vi "back_go_160607_85.vi"() -> ()   [LabVIEW 2015]
uses:
  <vilib>/NXT/Block Support/NXT_InputPort.ctl
  <vilib>/NXT/Block Support/NXT_OutputPort.ctl
  <vilib>/NXT/Dual Mode Library/Sensors/Light_On.vi
  <vilib>/NXT/Dual Mode Library/Sensors/Touch_Pressed.vi
  <vilib>/NXT/NXTIO Xnodes/NXTIONodeSubVIs/NXTMoveMotors.vi
  <vilib>/NXT/Dual Mode Library/Sensors/Sonar_cm.vi
  <vilib>/NXT/Dual Mode Library/Waits/Wait_Num.vi
  <vilib>/NXT/Subs/LVHSConnector.ctl
  <vilib>/NXT/NXTIO Xnodes/AddressXNode/NXTIOAddress.xnode
  <vilib>/NXT/NXTIO Xnodes/NXTIOXNode/NXTIO.xnode
  <vilib>/NXT/LegoClasses/BrickReference/BrickReference.lvclass
panel:
  in  "turn lefttC 2":i8=75
  in  "turn lefttB 2":i8=75
  in  "Go-ahead":i8=75
  out "check destance":i16(slide) scale=0.0..100.0
  in  "turn rightC":i8=75
  in  "turn rightB":i8=75
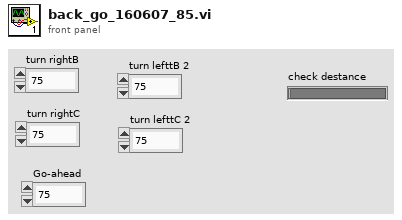
[diagram p1: front panel]
types:
  T1 = typedef "NXT_OutputPort.ctl" = u8
  T2 = typedef "NXT_InputPort.ctl" = u32
  T3 = typedef "LVHSConnector.ctl" = refnum<class "BrickReference.lvclass">
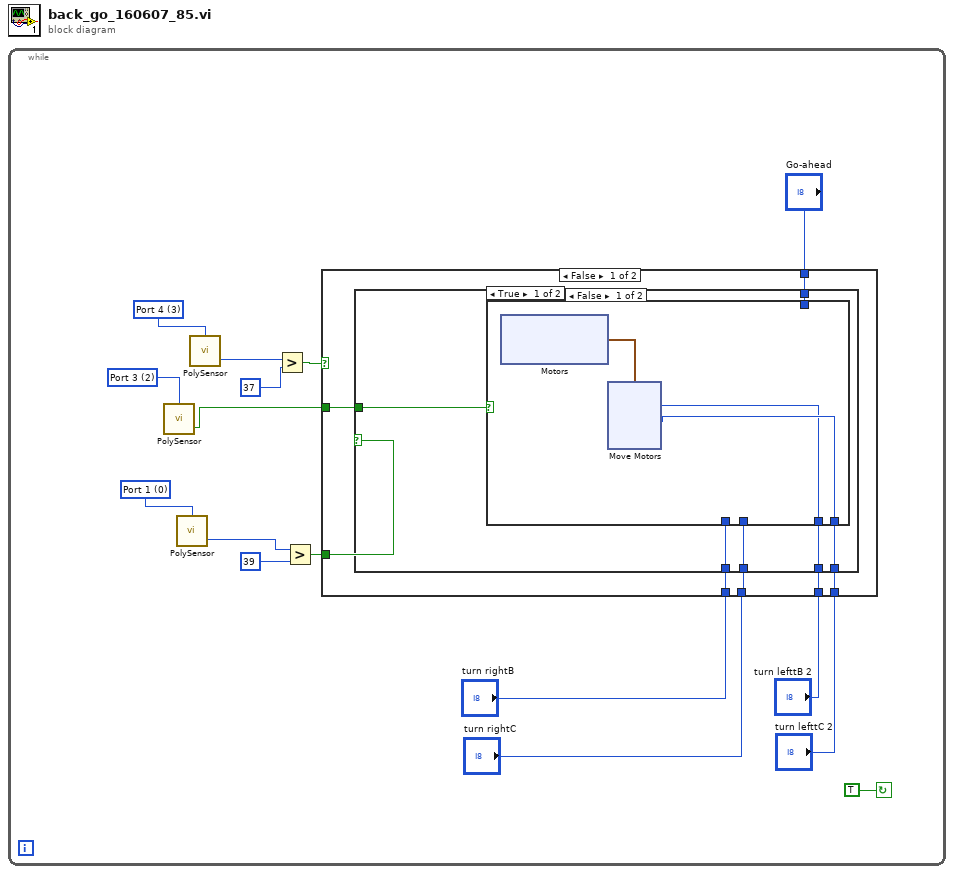
[diagram p0: block diagram]
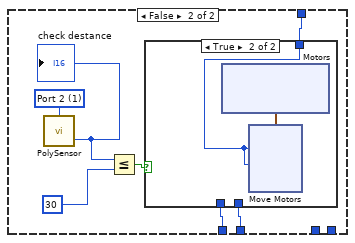
[diagram p2: hidden frame]
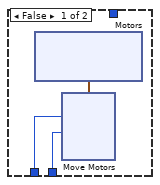
[diagram p3: hidden frame]
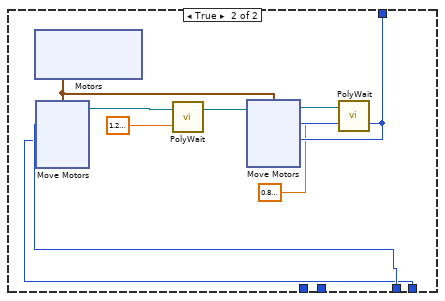
[diagram p4: hidden frame]
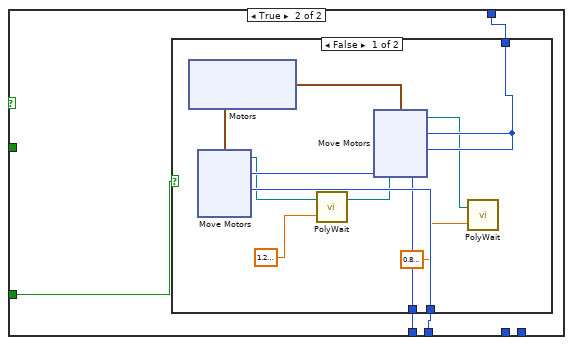
[diagram p5: hidden frame]
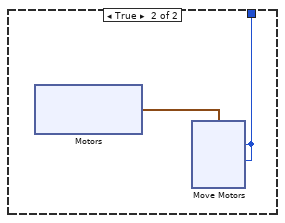
[diagram p6: hidden frame]
diagram:
  n1 = while {
    stop <- TRUE continue-if-true
    w1 = T2 2 items=["Port 1", "Port 2", "Port 3", "Port 4"] ("Port (Port 1)")
    w12 = T2 3 items=["Port 1", "Port 2", "Port 3", "Port 4"] ("Port (Port 3)")
    w11 = T2 0 items=["Port 1", "Port 2", "Port 3", "Port 4"] ("Port (Port 3)")
    n2 = call-poly <vilib>:"PolySensor.vi"("Port (Port 1)"=w1) -> ("Yes / No"=w2:bool)  [unwired: 2 in, 1 out]
    n3 = call-poly <vilib>:"PolySensor.vi"("Port (Port 3)"=w11) -> ("Scaled Value"=w13:i16)  [unwired: 2 in, 1 out]
    n4 = call-poly <vilib>:"PolySensor.vi"("Port (Port 3)"=w12) -> ("Scaled Value"=w15:i16)  [unwired: 2 in, 1 out]
    n5 = Greater?(x=w15, y=i16 37) -> (0:w10:bool)
    n6 = Greater?(x=w13, y=i16 39) -> (0:w9:bool)
    n7 = case shown="False" w10 {
      tunnel: w9 -> [w23 w101]
      tunnel: "turn rightB" -> [w22 w100]
      tunnel: "turn rightC" -> [w21 w99]
      tunnel: "Go-ahead" -> [w20 w98]
      tunnel: "turn lefttB 2" -> [w19 _]
      tunnel: "turn lefttC 2" -> [w18 _]
      tunnel: w2 -> [w17 _]
      frame False {
        n8 = case shown="False" w23 {
          tunnel: w22 -> [w29 _]
          tunnel: w21 -> [w28 _]
          tunnel: w20 -> [w27 w76]
          tunnel: w19 -> [w25 w80]
          tunnel: w18 -> [w24 w79]
          tunnel: w17 -> [w26 _]
          frame False {
            n9 = case shown="True" w26 {
              tunnel: w29 -> [_ w48]
              tunnel: w28 -> [_ w47]
              tunnel: w27 -> [_ w42]
              tunnel: w25 -> [w30 _]
              tunnel: w24 -> [w31 _]
              frame True {
                n10 = xnode "Motors"() -> ("Motor"=w32:cluster{"Port":T1, "Port":T1})
                n11 = xnode "Move Motors"("Power/Speed 2"=w31, "Power/Speed 1"=w30, "Motors"=w32) -> ()  [unwired: 1 in, 1 out]
              }
              frame False {
                w45 = T2 1 items=["Port 1", "Port 2", "Port 3", "Port 4"] ("Port (Port 4)")
                n12 = call-poly <vilib>:"PolySensor.vi"("Port (Port 4)"=w45) -> ("Distance (cm)"=w46:i16)  [unwired: 2 in, 1 out]
                "check destance" <- w46
                n13 = Less Or Equal?(x=w46, y=i16 30) -> (x <= y?=w43:bool)
                n14 = case shown="True" w43 {
                  tunnel: w48 -> [w50 _]
                  tunnel: w47 -> [w49 _]
                  tunnel: w42 -> [_ w61]
                  frame False {
                    n15 = xnode "Motors"() -> ("Motor"=w51:cluster{"Port":T1, "Port":T1})
                    n16 = xnode "Move Motors"("Power/Speed 2"=w49, "Power/Speed 1"=w50, "Motors"=w51) -> ()  [unwired: 1 in, 1 out]
                  }
                  frame True {
                    n17 = xnode "Motors"() -> ("Motor"=w62:cluster{"Port":T1, "Port":T1})
                    n18 = xnode "Move Motors"("Power/Speed 2"=w61, "Power/Speed 1"=w61, "Motors"=w62) -> ()  [unwired: 1 in, 1 out]
                  }
                }
              }
            }
          }
          frame True {
            n19 = xnode "Motors"() -> ("Motor"=w77:cluster{"Port":T1, "Port":T1})
            n20 = xnode "Move Motors"("Power/Speed 2"=w79, "Power/Speed 1"=w80, "Motors"=w77) -> ("NXT/EV3"=w78:T3)  [unwired: 1 in]
            n21 = call-poly <vilib>:"PolyWait.vi"("Time (1 sec)"=sgl 1.3, "NXT/EV3"=w78) -> ("NXT/EV3"=w75:T3)  [unwired: 2 in]
            n22 = xnode "Move Motors"("Power/Speed 2"=w76, "Power/Speed 1"=w76, "Motors"=w77, "NXT/EV3"=w75) -> ("NXT/EV3"=w74:T3)
            n23 = call-poly <vilib>:"PolyWait.vi"("Time (1 sec)"=sgl 0.8, "NXT/EV3"=w74) -> ()  [unwired: 2 in, 1 out]
          }
        }
      }
      frame True {
        n24 = case shown="False" w101 {
          tunnel: w100 -> [w109 _]
          tunnel: w99 -> [w110 _]
          tunnel: w98 -> [w107 w128]
          frame False {
            n25 = xnode "Motors"() -> ("Motor"=w108:cluster{"Port":T1, "Port":T1})
            n26 = xnode "Move Motors"("Power/Speed 2"=w110, "Power/Speed 1"=w109, "Motors"=w108) -> ("NXT/EV3"=w106:T3)  [unwired: 1 in]
            n27 = call-poly <vilib>:"PolyWait.vi"("Time (1 sec)"=sgl 1.3, "NXT/EV3"=w106) -> ("NXT/EV3"=w105:T3)  [unwired: 2 in]
            n28 = xnode "Move Motors"("Power/Speed 2"=w107, "Power/Speed 1"=w107, "Motors"=w108, "NXT/EV3"=w105) -> ("NXT/EV3"=w104:T3)
            n29 = call-poly <vilib>:"PolyWait.vi"("Time (1 sec)"=sgl 0.8, "NXT/EV3"=w104) -> ()  [unwired: 2 in, 1 out]
          }
          frame True {
            n30 = xnode "Motors"() -> ("Motor"=w129:cluster{"Port":T1, "Port":T1})
            n31 = xnode "Move Motors"("Power/Speed 2"=w128, "Power/Speed 1"=w128, "Motors"=w129) -> ()  [unwired: 1 in, 1 out]
          }
        }
      }
    }
  }
